vi "Example.vi"() -> (0 "error out":errorcluster)   [LabVIEW 2022 SP3, in "PythonWrapper.lvlib"]
uses:
  PythonWrapper.lvlib
  PythonWrapper/PythonWrapper.lvclass
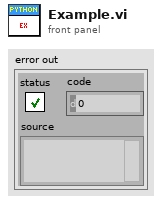
[diagram p1: front panel]
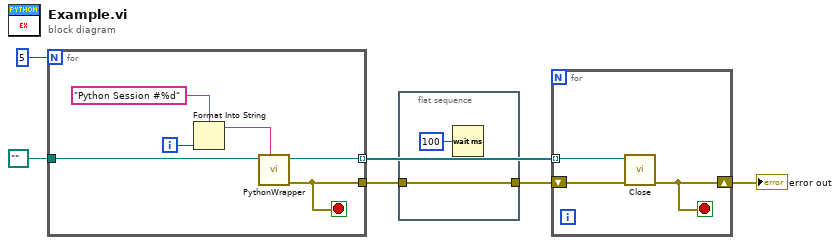
[diagram p0: block diagram]
diagram:
  n1 = for {
    N: 5 -> [_]
    tunnel: path "" ("ModulePath") -> [w12]
    tunnel: [w10] -> w1
    tunnel: [w9] -> w3 mode=indexing
    i -> [w11]
    stop <- w10 stop-if-true
    n2 = Format Into String(format string="Python Session #%d", w11) -> (resulting string=w7:string)  [unwired: 2 in, 1 out]
    n3 = call "PythonWrapper.vi"("SessionName"=w7, "ModulePath"=w12) -> ("error out"=w10:errorcluster, "PythonWrapper"=w9:refnum<class "PythonWrapper.lvclass">)  [unwired: 8 in]
  }
  n4 = flat-sequence {
    tunnel: [w14] -> w2
    tunnel: w1 -> [w14]
    frame #0 {
      n5 = Wait (ms)(milliseconds to wait=u32 100) -> ()  [unwired: 1 out]
    }
  }
  n6 = for {
    tunnel: w3 -> [w15] mode=indexing
    shift-right: [w17] -> w4
    shift-left: w2 -> [w16]
    stop <- w17 stop-if-true
    n7 = call-dynamic "Close.vi"("error in (no error)"=w16, "PythonWrapper in"=w15) -> ("error out"=w17:errorcluster)  [unwired: 9 in]
  }
  "error out" <- w4
